vi "Main interface.vi"() -> ()   [LabVIEW 2014]
panel:
  in  "Control stop":bool
  out "Control Running":bool
  in  "Tab Control":T1(tab)
  out "Analog Servo":dbl(knob) scale=0.0..360.0
  out "Stepper":dbl(knob) scale=0.0..360.0
  out "PWM Servo":dbl(knob) scale=0.0..360.0
  in  "Set Point Pot":dbl(knob) scale=0.0..360.0
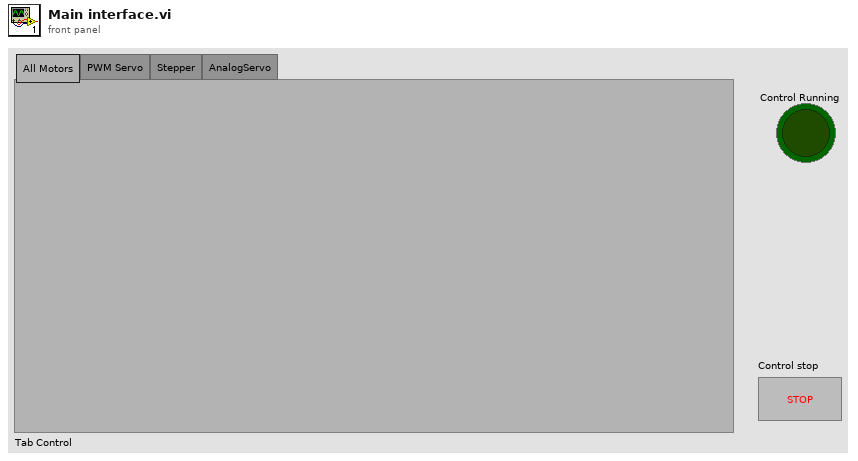
[diagram p1: front panel]
types:
  T1 = enum32{"All Motors", "PWM Servo", "Stepper", "AnalogServo"}
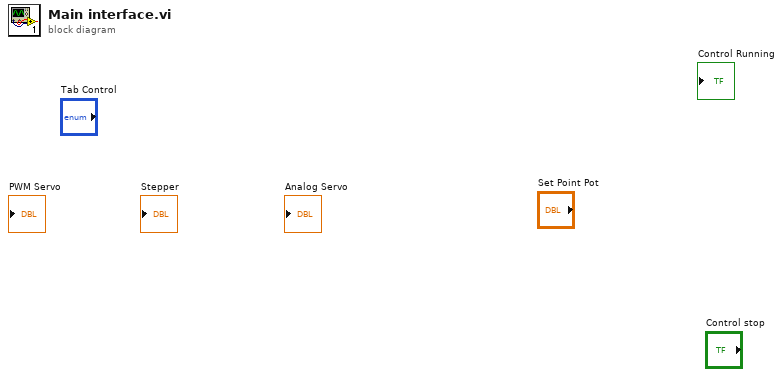
[diagram p0: block diagram]
diagram:
